vi "Destroy.vi"(8 "Error In":errorcluster, 11 "reference in":refnum<class "SedanCarFactory.lvclass">) -> (0 "Error Out":errorcluster, 3 "reference out":refnum<class "SedanCarFactory.lvclass">)   [LabVIEW 2024, in "SedanCarFactory.lvclass"]
uses:
  SedanCarFactory.lvclass
  SedanCarFactory.lvclass/SedanCarFactory.ctl
  CarFactory/CarFactory.lvclass
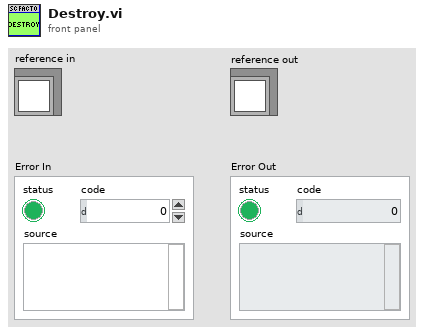
[diagram p1: front panel]
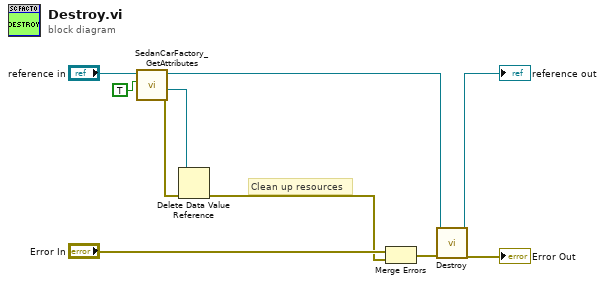
[diagram p0: block diagram]
diagram:
  # "Clean up resources"
  n1 = call "SedanCarFactory_GetAttributes.vi"("OnlyGetDvrReference(False)"=TRUE, "reference in"="reference in") -> ("Error Out"=w8:errorcluster, "DataRef"=w6:refnum<data-value>, "reference out"=w7:refnum<class "SedanCarFactory.lvclass">)  [unwired: 6 in, 1 out]
  n2 = Delete Data Value Reference(data value reference=w6, error in=w8) -> (error out=w4:errorcluster)  [unwired: 1 out]
  n3 = Merge Errors("Error In", w4) -> (w10:errorcluster)
  n4 = call-parent "Destroy.vi"("Error In"=w10, "reference in"=w7) -> ("Error Out"=→"Error Out":errorcluster, "reference out"=→"reference out":refnum<class "SedanCarFactory.lvclass">)  [unwired: 8 in]
